vi "consol_0001.vi"() -> ()   [LabVIEW 2012]
uses:
  <vilib>/Utility/file.llb/Write To Spreadsheet File (DBL).vi
panel:
  in  "Test":bool
  out "Old Exposure":u32
  out "XY Graph":cluster{dbl[], "framePixelsBuffer":dbl[]}(graph)
  in  "Norm":bool=TRUE
  out "string Out":string
  in  "numOfScans":u16=4
  in  "timeOfExposure (32 bit)":u32=50
  out "statusFlags":u8
  in  "save":bool
  in  "stop":bool
  in  "numOfFrame":u16=65535 format="%x"
  # "in 10 microseconds units"
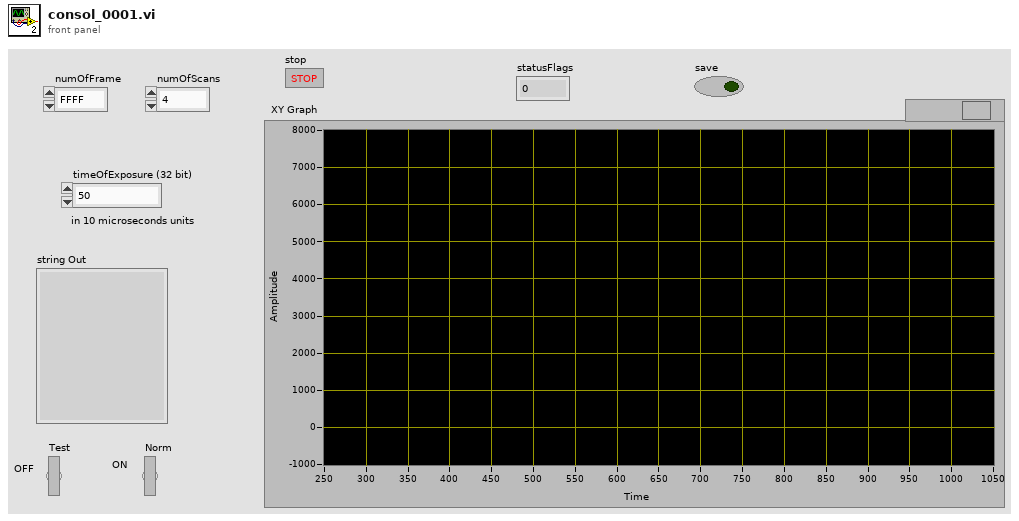
[diagram p1: front panel]
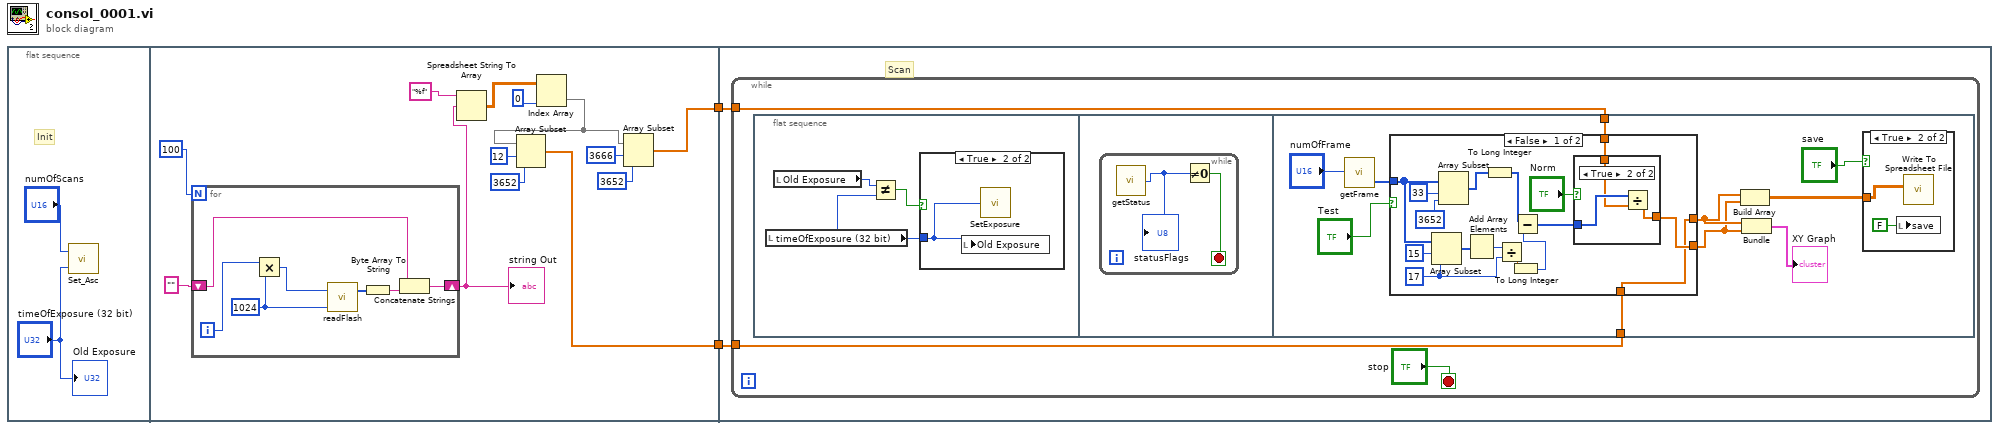
[diagram p0: block diagram]
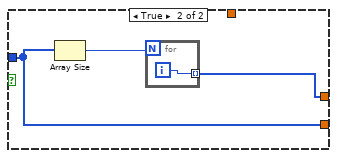
[diagram p5: hidden frame]
diagram:
  n1 = flat-sequence {
    tunnel: [w7] -> w2
    tunnel: [w6] -> w1
    tunnel: w2 -> [w26]
    tunnel: w1 -> [w25]
    frame #0 {
      # "Init"
      n2 = call "Set_Asc.vi"("timeOfExposure (32 bit)"="timeOfExposure (32 bit)", "numOfScans"="numOfScans") -> ()  [unwired: 1 in]
      "Old Exposure" <- "timeOfExposure (32 bit)"
    }
    frame #1 {
      n3 = for {
        N: 100 -> [_]
        shift-right: [w19] -> w5
        shift-left: "" -> [w21]
        i -> [w22]
        w23 = u16 1024 ("bytesToRead")
        n4 = Multiply(x=w22, y=w23) -> (x*y=w18:i32)
        n5 = call "readFlash.vi"("bytesToRead"=w23, "offset"=w18) -> ("buffer"=w24:u8[])  [unwired: 1 out]
        n6 = Byte Array To String(unsigned byte array=w24) -> (string=w20:string)
        n7 = Concatenate Strings(w21, w20) -> (w19:string)
      }
      "string Out" <- w5
      n8 = Spreadsheet String To Array(format string="%f", spreadsheet string=w5) -> (array=w10:dbl[][])  [unwired: 2 in]
      n9 = Index Array(array=w10, index (col)=0 ("disabled index (col)")) -> (element=w8:dbl[])  [unwired: 1 in]
      n10 = Array Subset(array=w8, index=12, length=3652) -> (w6:dbl[])
      n11 = Array Subset(array=w8, index=3666, length=3652) -> (w7:dbl[])
    }
    frame #2 {
      # "Scan"
      n12 = while {
        tunnel: w26 -> [w28]
        tunnel: w25 -> [w27]
        stop <- "stop" stop-if-true
        n13 = flat-sequence {
          tunnel: w28 -> [w41]
          tunnel: w27 -> [w40]
          frame #0 {
            n14 = local read "timeOfExposure (32 bit)"() -> (w30:u32)
            n15 = local read "Old Exposure"() -> (w32:u32)
            n16 = Not Equal?(x=w32, y=w30) -> (x != y?=w31:bool)
            n17 = case shown="True" w31 {
              tunnel: w30 -> [_ w33]
              frame False {
              }
              frame True {
                n18 = local write "Old Exposure"(w33) -> ()
                n19 = call "SetExposure.vi"("Exposure"=w33) -> ()  [unwired: 1 out]
              }
            }
          }
          frame #1 {
            n20 = while {
              stop <- w35 stop-if-true
              n21 = call "getStatus.vi"() -> ("statusFlags"=w34:u8)  [unwired: 2 out]
              "statusFlags" <- w34
              n22 = Not Equal To 0?(x=w34) -> (x != 0?=w35:bool)
            }
          }
          frame #2 {
            n23 = call "getFrame.vi"("numOfFrame"="numOfFrame") -> ("framePixelsBuffer"=w44:u16[])  [unwired: 1 out]
            n24 = case shown="False" "Test" {
              tunnel: w44 -> [w61 w69]
              tunnel: w41 -> [w50 _]
              tunnel: w40 -> [w48 _]
              tunnel: [w49 w69] -> w37
              tunnel: [w48 w70] -> w38
              frame False {
                w57 = 17 ("length")
                n25 = Array Subset(array=w61, index=15, length=w57) -> (w59:u16[])
                n26 = Array Subset(array=w61, index=33, length=3652) -> (w56:u16[])
                n27 = Add Array Elements(numeric array=w59) -> (sum=w58:u16)
                n28 = To Long Integer(number=w56) -> (32bit integer=w55:i32[])
                n29 = Divide(x=w58, y=w57) -> (x/y=w54:dbl)
                n30 = To Long Integer(number=w54) -> (32bit integer=w53:i32)
                n31 = Subtract(x=w55, y=w53) -> (x-y=w51:i32[])
                n32 = case shown="True" "Norm" {
                  tunnel: w51 -> [w64 w67]
                  tunnel: w50 -> [_ w65]
                  tunnel: [w64 w66] -> w49
                  frame False {
                  }
                  frame True {
                    n33 = Divide(x=w67, y=w65) -> (x/y=w66:dbl[])
                  }
                }
              }
              frame True {
                n34 = Array Size(array=w69) -> (size(s)=w68:i32)
                n35 = for {
                  N: w68 -> [_]
                  tunnel: [w71] -> w70 mode=indexing
                  i -> [w71]
                }
              }
            }
            n36 = Build Array(w38, w37) -> (w36:dbl[][])
            n37 = Bundle(w38, "framePixelsBuffer"=w37) -> (→"XY Graph":cluster{dbl[], "framePixelsBuffer":dbl[]})  [unwired: 1 in]
            n38 = case shown="True" "save" {
              tunnel: w36 -> [_ w46]
              frame False {
              }
              frame True {
                n39 = local write "save"(FALSE ("save")) -> ()
                n40 = call-poly <vilib>:"Write To Spreadsheet File.vi"("2D data"=w46) -> ()  [unwired: 7 in, 1 out]
              }
            }
          }
        }
      }
    }
  }
